vi "Add Tags.vi"(8 "error in (no error)":errorcluster, 10 "Tag":string[](array[string]), 11 "Tag Tree Helper In":refnum<class "Tag Tree Helper.lvclass">) -> (0 "error out":errorcluster, 3 "Tag Tree Helper Out":refnum<class "Tag Tree Helper.lvclass">)   [LabVIEW 2020, in "Tag Tree Helper.lvclass"]
uses:
  Tag Tree Helper.lvclass
panel:
  in  "Child Text":string[][](array[string])
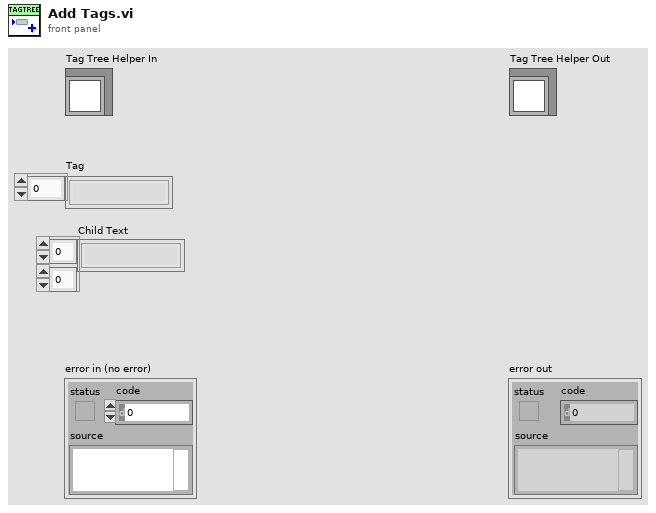
[diagram p1: front panel]
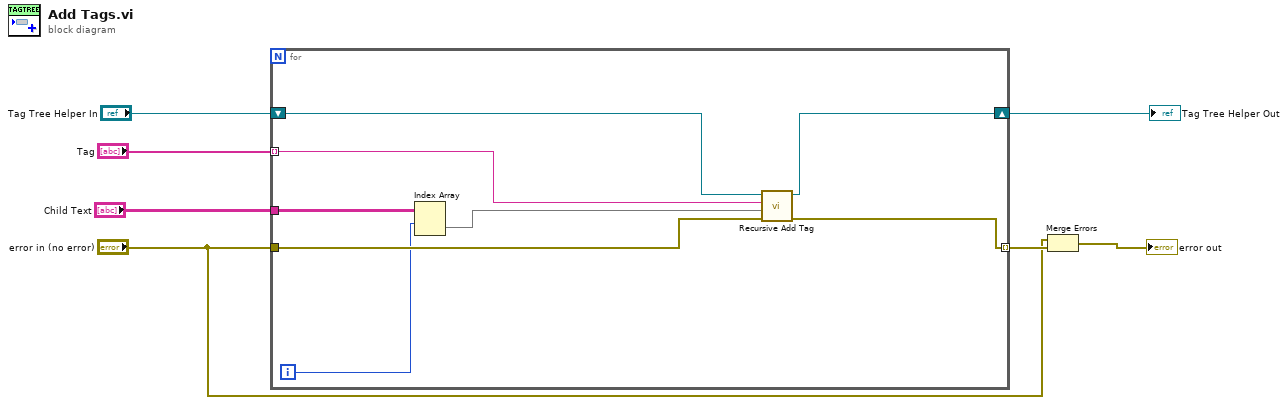
[diagram p0: block diagram]
diagram:
  n1 = for {
    tunnel: "Tag" -> [w15] mode=indexing
    shift-right: [w11] -> w5
    shift-left: "Tag Tree Helper In" -> [w12]
    tunnel: "error in (no error)" -> [w14]
    tunnel: [w13] -> w4 mode=indexing
    tunnel: "Child Text" -> [w8]
    i -> [w10]
    n2 = Index Array(array=w8, index (row)=w10) -> (element=w9:string[])  [unwired: 1 in]
    n3 = call "Recursive Add Tag.vi"("error in (no error)"=w14, "Child Text"=w9, "Tag"=w15, "Tag Tree Helper In"=w12) -> ("error out"=w13:errorcluster, "Tag Tree Helper Out"=w11:refnum<class "Tag Tree Helper.lvclass">)  [unwired: 6 in]
  }
  "Tag Tree Helper Out" <- w5
  n4 = Merge Errors("error in (no error)", w4) -> (→"error out":errorcluster)
